vi "ValidateCharacters.vi"(11 "Subsystem Name (optional)":string) -> (3 "Validated characters":string)   [LabVIEW 2021, in "smo.lvlib" / "Registry-SMO.lvclass"]
uses:
  Registry-SMO.lvclass
  Registry-SMO.lvclass/Registry-SMO.ctl
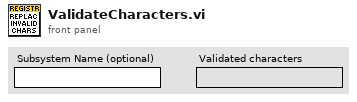
[diagram p1: front panel]
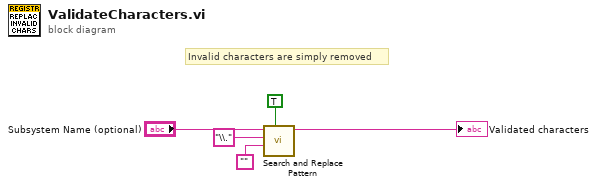
[diagram p0: block diagram]
diagram:
  # "Invalid characters are simply removed"
  n1 = call <vilib>:"Search and Replace Pattern.vi"("string"="Subsystem Name (optional)", "regular expression (\"\")"="\\." ("regular expression (\"\")"), "replace string (\"\")"="" ("regular expression (\"\")"), "replace all? (F)"=TRUE) -> ("result string"=→"Validated characters":string)  [unwired: 1 in, 1 out]
